vi "Rapidox parse.vi"(10 "RapidoxOutput":u8[](array[numeric])=[100, 50, 46, 48, 50, 52, 69, 43, 48, 53, 44, 49, 46, 49, 51, 54, 69, 43, 48, 49, 44, 49, 46, 48, 49, 53, 69, 43, 48, 48, 44, 49, 56, 58, 49, 49, 58, 49, 56, 44, 50, 56, 47, 48, 57, 47, 49, 49, 44, 44, 48, 13, 10, 0]) -> (2 "O2 %":dbl)   [LabVIEW 2014]
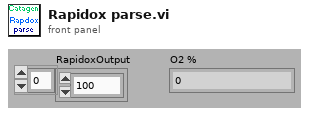
[diagram p1: front panel]
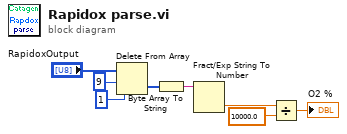
[diagram p0: block diagram]
diagram:
  n1 = Delete From Array(array="RapidoxOutput", length=9, index=1) -> (deleted portion=w5:u8[])  [unwired: 1 out]
  n2 = Byte Array To String(unsigned byte array=w5) -> (string=w4:string)
  n3 = Fract/Exp String To Number(string=w4) -> (number=w3:dbl)  [unwired: 3 in, 1 out]
  n4 = Divide(x=w3, y=10000.0) -> (x/y=→"O2 %":dbl)
